vi "AUTON_Index.vi"(0 "Auton Array":dbl[][](array[numeric]), 5 "MeasuredHeading":dbl, 7 "LeftEncoder":dbl, 9 "RightEncoder":dbl) -> ()   [LabVIEW 2012]
uses:
  Robot Global Data.vi
panel:
  out "Right Kicker":dbl
  out "Left Flipper":dbl
  out "Right Flipper":dbl
  out "Shooter Wheel B":dbl
  out "Shooter Wheel F":dbl
  out "Shooter Elevation":dbl
  out "Left Kicker":dbl
  out "Right Drive":dbl
  out "Left Drive":dbl
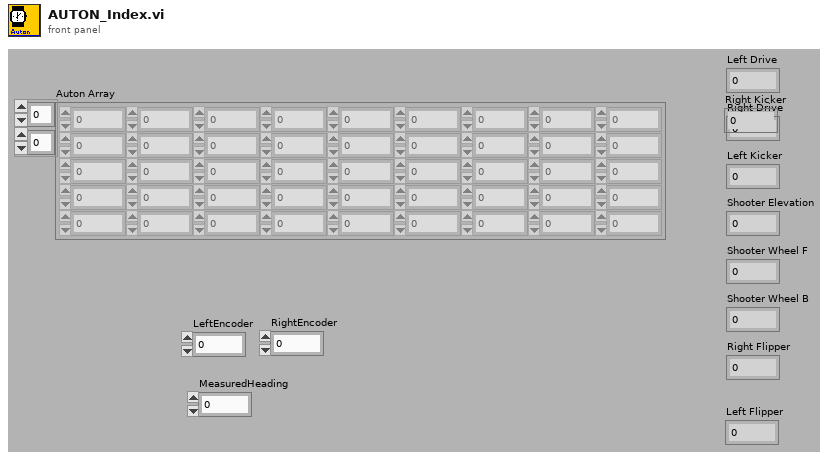
[diagram p1: front panel]
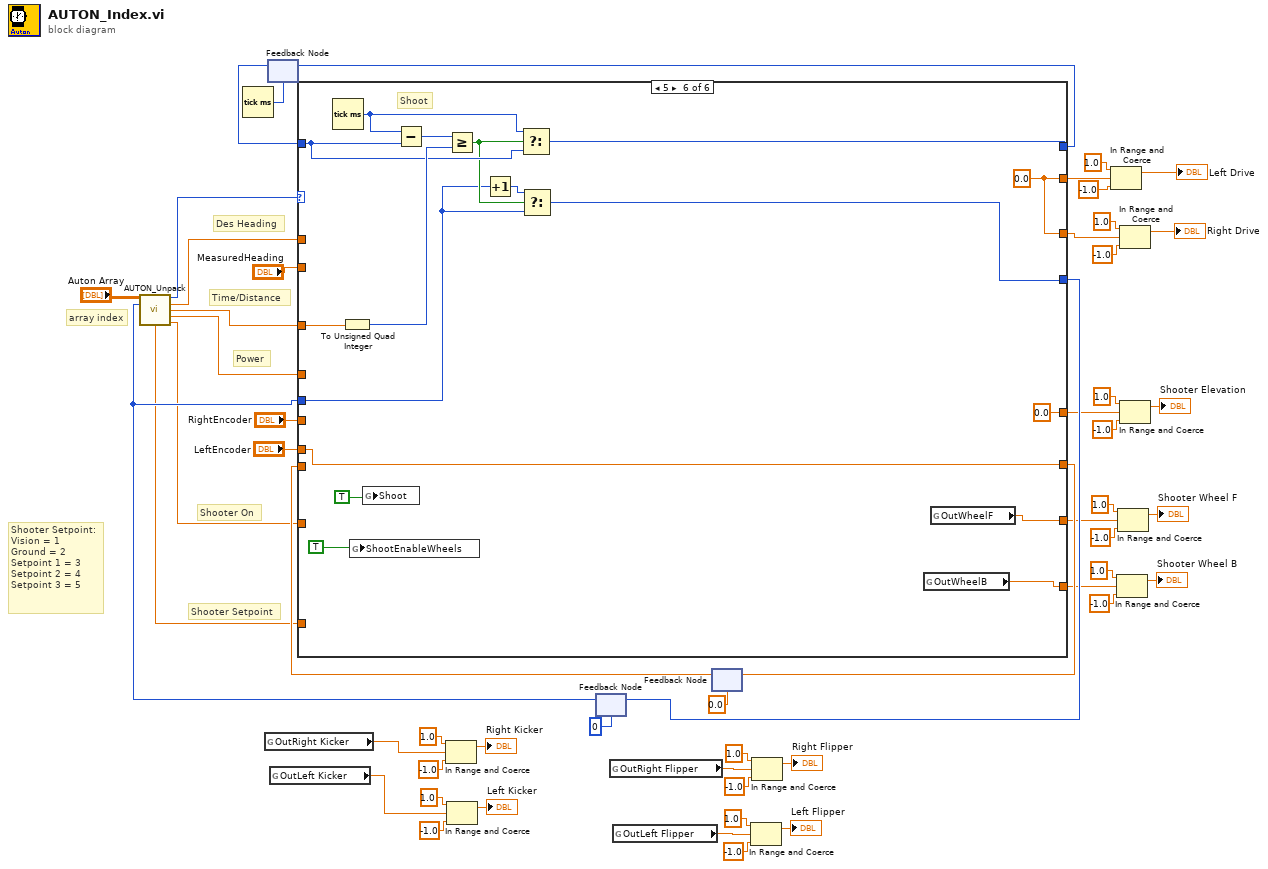
[diagram p0: block diagram]
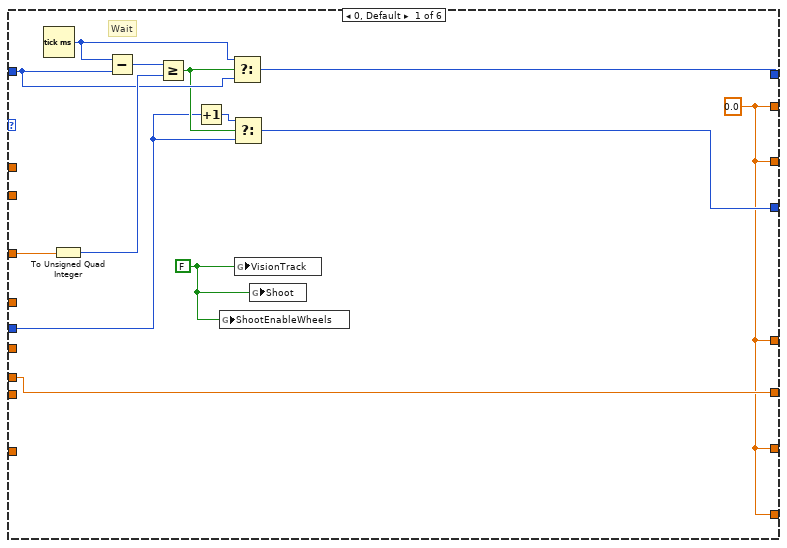
[diagram p2: hidden frame]
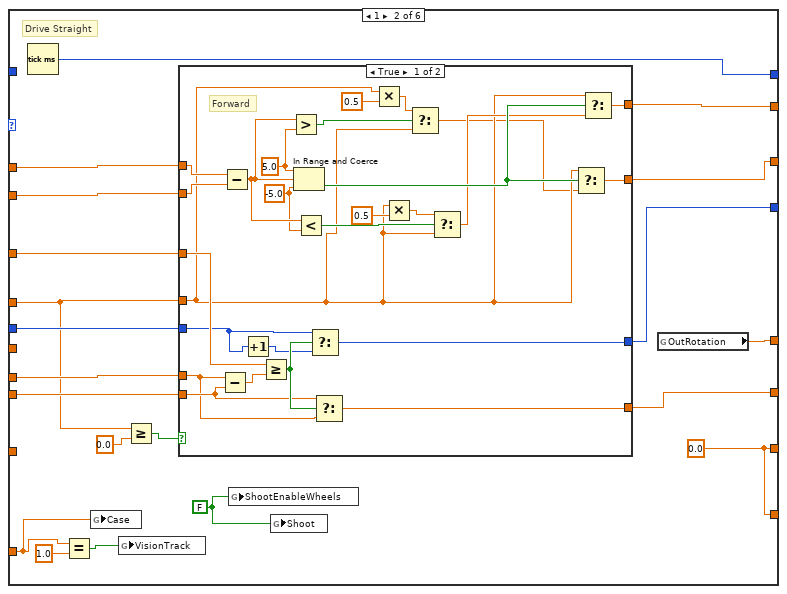
[diagram p3: hidden frame]
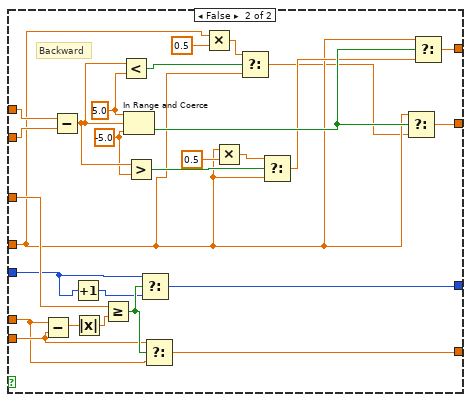
[diagram p4: hidden frame]
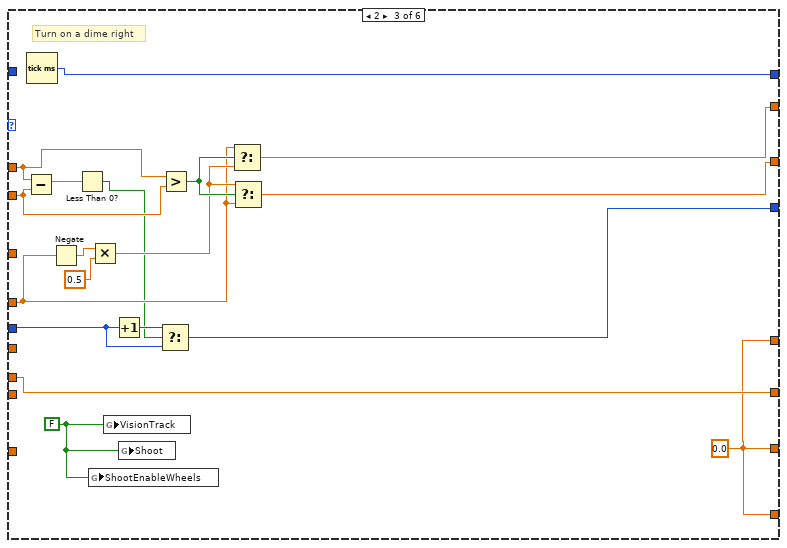
[diagram p5: hidden frame]
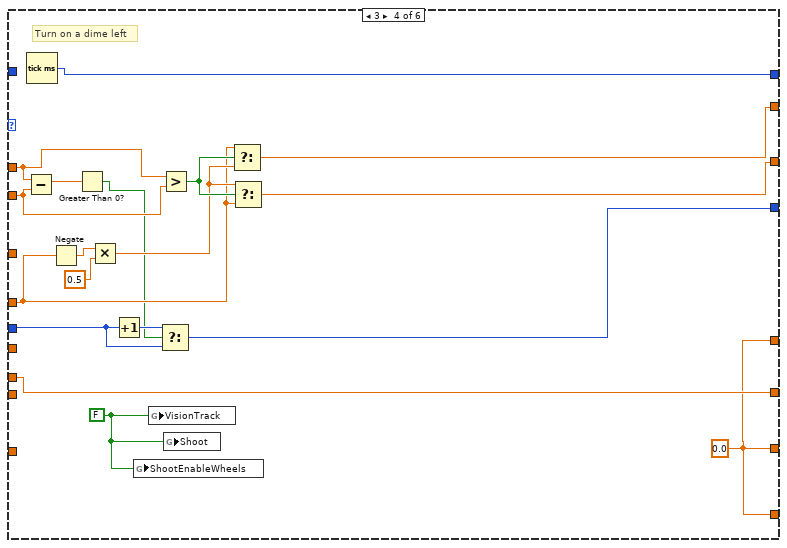
[diagram p6: hidden frame]
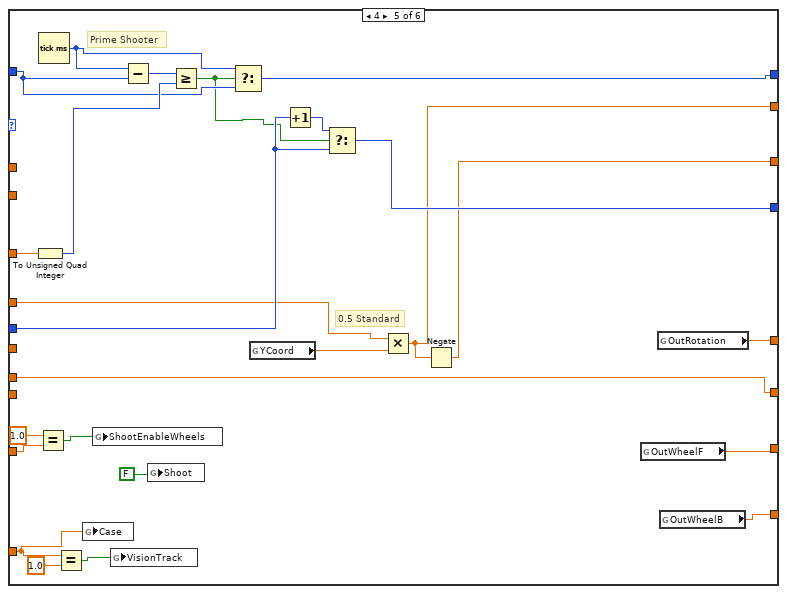
[diagram p7: hidden frame]
diagram:
  # "Shooter Setpoint:\nVision = 1\nGround = 2\nSetpoint 1 = 3\nSetpoint 2 = 4\nSetpoint 3 = 5"
  # "Shooter On"
  # "Shooter Setpoint"
  # "Des Heading"
  # "Time/Distance"
  # "Power"
  # "array index"
  n1 = Tick Count (ms)() -> (millisecond timer value=w52:u32)
  n2 = global read "Robot Global Data.vi" "OutRight Kicker"() -> (w1:dbl)
  n3 = feedback #1(w52) -> (w54:u32)
  n4 = global read "Robot Global Data.vi" "OutLeft Kicker"() -> (w2:dbl)
  n5 = In Range and Coerce(upper limit=1.0, x=w1, lower limit=-1.0) -> (coerced(x)=→"Right Kicker":dbl)  [unwired: 1 out]
  n6 = In Range and Coerce(upper limit=1.0, x=w2, lower limit=-1.0) -> (coerced(x)=→"Left Kicker":dbl)  [unwired: 1 out]
  n7 = feedback #2(0) -> (w31:i32)
  n8 = call "AUTON_Unpack.vi"("all rows"="Auton Array", "Index"=w31) -> ("Primitive ID"=w35:i16, "Desired Heading"=w33:dbl, "Time/Distance"=w32:dbl, "Power"=w34:dbl, "Shooter Setpoint"=w29:dbl, "Shooter Speed"=w30:dbl)  [unwired: 6 in, 2 out]
  n9 = global read "Robot Global Data.vi" "OutRight Flipper"() -> (w10:dbl)
  n10 = global read "Robot Global Data.vi" "OutLeft Flipper"() -> (w9:dbl)
  n11 = feedback #3(0.0) -> (w37:dbl)
  n12 = case shown="5" w35 {
    tunnel: [w60 w86 w154 w172 w201 w211] -> w40
    tunnel: w31 -> [w61 w81 w157 w175 w192 w212]
    tunnel: [w68 w78 w159 w177 w190 w219] -> w42
    tunnel: w54 -> [w65 _ _ _ w191 w216]
    tunnel: w32 -> [w59 w87 _ _ w193 w210]
    tunnel: w33 -> [_ w85 w152 w170 _ _]
    tunnel: [w56 w83 w155 w173 w186 w209] -> w50
    tunnel: [w56 w82 w156 w174 w185 w209] -> w43
    tunnel: w34 -> [_ w77 w146 w164 w187 _]
    tunnel: "LeftEncoder" -> [w57 w79 w153 w171 w202 w207]
    tunnel: "MeasuredHeading" -> [_ w84 w151 w169 _ _]
    tunnel: "RightEncoder" -> [_ _ _ _ _ _]
    tunnel: w37 -> [_ w80 _ _ _ _]
    tunnel: [w57 w88 w153 w171 w202 w207] -> w36
    tunnel: w30 -> [_ _ _ _ w182 _]
    tunnel: w29 -> [_ w71 _ _ w197 _]
    tunnel: [w56 w69 w143 w160 w178 w203] -> w13
    tunnel: [w56 w69 w143 w160 w179 w204] -> w12
    tunnel: [w56 w70 w143 w160 w189 0.0 ("ShootOutElev")] -> w11
    frame 0, Default {
      w58 = FALSE ("ShootTrackEnable")
      w56 = 0.0 ("Numeric")
      # "Wait"
      n13 = Tick Count (ms)() -> (millisecond timer value=w64:u32)
      n14 = To Unsigned Quad Integer(1:w59) -> (0:w66:u64)
      n15 = Subtract(x=w64, y=w65) -> (x-y=w67:u32)
      n16 = Greater Or Equal?(x=w67, y=w66) -> (x >= y?=w63:bool)
      n17 = Increment(x=w61) -> (x+1=w62:i32)
      n18 = global write "Robot Global Data.vi" "ShootEnableWheels"(w58) -> ()
      n19 = Select(t=w64, s=w63, f=w65) -> (s? t:f=w68:u32)
      n20 = Select(t=w62, s=w63, f=w61) -> (s? t:f=w60:i32)
      n21 = global write "Robot Global Data.vi" "VisionTrack"(w58) -> ()
      n22 = global write "Robot Global Data.vi" "Shoot"(w58) -> ()
    }
    frame 1 {
      w74 = FALSE ("ShootTrackEnable")
      w69 = 0.0 ("Numeric")
      # "Drive Straight"
      n23 = Tick Count (ms)() -> (millisecond timer value=w78:u32)
      n24 = Equal?(x=w71, y=1.0) -> (x = y?=w72:bool)
      n25 = global write "Robot Global Data.vi" "Case"(w71) -> ()
      n26 = global write "Robot Global Data.vi" "VisionTrack"(w72) -> ()
      n27 = Greater Or Equal?(x=w77, y=0.0) -> (x >= y?=w75:bool)
      n28 = case shown="True" w75 {
        tunnel: [w114 w141] -> w88
        tunnel: w87 -> [w112 w140]
        tunnel: [w110 w138] -> w86
        tunnel: w85 -> [w109 w137]
        tunnel: w84 -> [w108 w136]
        tunnel: [w106 w134] -> w83
        tunnel: [w105 w133] -> w82
        tunnel: w77 -> [w94 w122]
        tunnel: w81 -> [w91 w119]
        tunnel: w80 -> [w90 w118]
        tunnel: w79 -> [w89 w117]
        frame True {
          w102 = -5.0 ("lower limit")
          w104 = 5.0 ("upper limit")
          # "Forward"
          n29 = Subtract(x=w89, y=w90) -> (x-y=w113:dbl)
          n30 = Subtract(x=w109, y=w108) -> (x-y=w103:dbl)
          n31 = Increment(x=w91) -> (x+1=w92:i32)
          n32 = Greater Or Equal?(x=w112, y=w113) -> (x >= y?=w111:bool)
          n33 = Greater?(x=w103, y=w104) -> (0:w97:bool)
          n34 = In Range and Coerce(upper limit=w104, x=w103, lower limit=w102) -> (In Range?=w107:bool)  [unwired: 1 out]
          n35 = Less?(x=w103, y=w102) -> (x < y?=w101:bool)
          n36 = Select(t=w91, s=w111, f=w92) -> (s? t:f=w110:i32)
          n37 = Select(t=w90, s=w111, f=w89) -> (s? t:f=w114:dbl)
          n38 = Multiply(x=w94, y=0.5) -> (x*y=w96:dbl)
          n39 = Multiply(x=w94, y=0.5) -> (x*y=w99:dbl)
          n40 = Select(t=w96, s=w97, f=w94) -> (s? t:f=w93:dbl)
          n41 = Select(t=w99, s=w101, f=w94) -> (s? t:f=w98:dbl)
          n42 = Select(t=w94, s=w107, f=w93) -> (s? t:f=w105:dbl)
          n43 = Select(t=w94, s=w107, f=w98) -> (s? t:f=w106:dbl)
        }
        frame False {
          w130 = -5.0 ("lower limit")
          w132 = 5.0 ("upper limit")
          # "Backward"
          n44 = Subtract(x=w117, y=w118) -> (x-y=w115:dbl)
          n45 = Subtract(x=w137, y=w136) -> (x-y=w131:dbl)
          n46 = Increment(x=w119) -> (x+1=w120:i32)
          n47 = Absolute Value(x=w115) -> (abs(x)=w116:dbl)
          n48 = Greater Or Equal?(x=w140, y=w116) -> (x >= y?=w139:bool)
          n49 = Less?(x=w131, y=w132) -> (x < y?=w125:bool)
          n50 = In Range and Coerce(upper limit=w132, x=w131, lower limit=w130) -> (In Range?=w135:bool)  [unwired: 1 out]
          n51 = Greater?(x=w131, y=w130) -> (0:w129:bool)
          n52 = Select(t=w119, s=w139, f=w120) -> (s? t:f=w138:i32)
          n53 = Select(t=w118, s=w139, f=w117) -> (s? t:f=w141:dbl)
          n54 = Multiply(x=w122, y=0.5) -> (x*y=w124:dbl)
          n55 = Multiply(x=w122, y=0.5) -> (x*y=w127:dbl)
          n56 = Select(t=w124, s=w125, f=w122) -> (s? t:f=w121:dbl)
          n57 = Select(t=w127, s=w129, f=w122) -> (s? t:f=w126:dbl)
          n58 = Select(t=w122, s=w135, f=w121) -> (s? t:f=w133:dbl)
          n59 = Select(t=w122, s=w135, f=w126) -> (s? t:f=w134:dbl)
        }
      }
      n60 = global write "Robot Global Data.vi" "ShootEnableWheels"(w74) -> ()
      n61 = global write "Robot Global Data.vi" "Shoot"(w74) -> ()
      n62 = global read "Robot Global Data.vi" "OutRotation"() -> (w70:dbl)
    }
    frame 2 {
      w142 = FALSE ("ShootTrackEnable")
      w143 = 0.0 ("Numeric")
      # "Turn on a dime right"
      n63 = Subtract(x=w152, y=w151) -> (x-y=w145:dbl)
      n64 = Tick Count (ms)() -> (millisecond timer value=w159:u32)
      n65 = Negate(x=w146) -> (-x=w149:dbl)
      n66 = Less Than 0?(x=w145) -> (x < 0?=w144:bool)
      n67 = global write "Robot Global Data.vi" "ShootEnableWheels"(w142) -> ()
      n68 = Multiply(x=w149, y=0.5) -> (x*y=w147:dbl)
      n69 = global write "Robot Global Data.vi" "VisionTrack"(w142) -> ()
      n70 = Increment(x=w157) -> (x+1=w158:i32)
      n71 = global write "Robot Global Data.vi" "Shoot"(w142) -> ()
      n72 = Select(t=w158, s=w144, f=w157) -> (s? t:f=w154:i32)
      n73 = Greater?(x=w152, y=w151) -> (0:w150:bool)
      n74 = Select(t=w146, s=w150, f=w147) -> (s? t:f=w155:dbl)
      n75 = Select(t=w147, s=w150, f=w146) -> (s? t:f=w156:dbl)
    }
    frame 3 {
      w161 = FALSE ("ShootTrackEnable")
      w160 = 0.0 ("Numeric")
      # "Turn on a dime left"
      n76 = Subtract(x=w170, y=w169) -> (x-y=w163:dbl)
      n77 = Tick Count (ms)() -> (millisecond timer value=w177:u32)
      n78 = Negate(x=w164) -> (-x=w167:dbl)
      n79 = Greater Than 0?(x=w163) -> (x > 0?=w162:bool)
      n80 = Multiply(x=w167, y=0.5) -> (x*y=w165:dbl)
      n81 = Increment(x=w175) -> (x+1=w176:i32)
      n82 = global write "Robot Global Data.vi" "ShootEnableWheels"(w161) -> ()
      n83 = global write "Robot Global Data.vi" "VisionTrack"(w161) -> ()
      n84 = Select(t=w176, s=w162, f=w175) -> (s? t:f=w172:i32)
      n85 = Greater?(x=w170, y=w169) -> (0:w168:bool)
      n86 = global write "Robot Global Data.vi" "Shoot"(w161) -> ()
      n87 = Select(t=w164, s=w168, f=w165) -> (s? t:f=w173:dbl)
      n88 = Select(t=w165, s=w168, f=w164) -> (s? t:f=w174:dbl)
    }
    frame 4 {
      # "0.5 Standard"
      # "Prime Shooter"
      n89 = To Unsigned Quad Integer(1:w193) -> (0:w195:u64)
      n90 = Equal?(x=1.0, y=w182) -> (x = y?=w180:bool)
      n91 = Tick Count (ms)() -> (millisecond timer value=w194:u32)
      n92 = Equal?(x=w197, y=1.0) -> (x = y?=w198:bool)
      n93 = global write "Robot Global Data.vi" "Case"(w197) -> ()
      n94 = global write "Robot Global Data.vi" "ShootEnableWheels"(w180) -> ()
      n95 = global write "Robot Global Data.vi" "VisionTrack"(w198) -> ()
      n96 = Subtract(x=w194, y=w191) -> (x-y=w196:u32)
      n97 = global write "Robot Global Data.vi" "Shoot"(FALSE ("Shoot")) -> ()
      n98 = Greater Or Equal?(x=w196, y=w195) -> (x >= y?=w188:bool)
      n99 = Select(t=w194, s=w188, f=w191) -> (s? t:f=w190:u32)
      n100 = global read "Robot Global Data.vi" "YCoord"() -> (w184:dbl)
      n101 = Increment(x=w192) -> (x+1=w200:i32)
      n102 = Select(t=w200, s=w188, f=w192) -> (s? t:f=w201:i32)
      n103 = Multiply(x=w187, y=w184) -> (x*y=w186:dbl)
      n104 = Negate(x=w186) -> (-x=w185:dbl)
      n105 = global read "Robot Global Data.vi" "OutWheelF"() -> (w179:dbl)
      n106 = global read "Robot Global Data.vi" "OutRotation"() -> (w189:dbl)
      n107 = global read "Robot Global Data.vi" "OutWheelB"() -> (w178:dbl)
    }
    frame 5 {
      w209 = 0.0 ("Numeric")
      # "Shoot"
      n108 = Tick Count (ms)() -> (millisecond timer value=w215:u32)
      n109 = To Unsigned Quad Integer(1:w210) -> (0:w217:u64)
      n110 = global write "Robot Global Data.vi" "ShootEnableWheels"(TRUE ("ShootEnableWheels")) -> ()
      n111 = global write "Robot Global Data.vi" "Shoot"(TRUE ("Shoot")) -> ()
      n112 = Subtract(x=w215, y=w216) -> (x-y=w218:u32)
      n113 = Greater Or Equal?(x=w218, y=w217) -> (x >= y?=w214:bool)
      n114 = Increment(x=w212) -> (x+1=w213:i32)
      n115 = Select(t=w215, s=w214, f=w216) -> (s? t:f=w219:u32)
      n116 = Select(t=w213, s=w214, f=w212) -> (s? t:f=w211:i32)
      n117 = global read "Robot Global Data.vi" "OutWheelB"() -> (w203:dbl)
      n118 = global read "Robot Global Data.vi" "OutWheelF"() -> (w204:dbl)
    }
  }
  n119 = feedback-in #1(w42) -> ()
  n120 = feedback-in #2(w40) -> ()
  n121 = feedback-in #3(w36) -> ()
  n122 = In Range and Coerce(upper limit=1.0, x=w9, lower limit=-1.0) -> (coerced(x)=→"Left Flipper":dbl)  [unwired: 1 out]
  n123 = In Range and Coerce(upper limit=1.0, x=w10, lower limit=-1.0) -> (coerced(x)=→"Right Flipper":dbl)  [unwired: 1 out]
  n124 = In Range and Coerce(upper limit=1.0, x=w50, lower limit=-1.0) -> (coerced(x)=→"Left Drive":dbl)  [unwired: 1 out]
  n125 = In Range and Coerce(upper limit=1.0, x=w13, lower limit=-1.0) -> (coerced(x)=→"Shooter Wheel B":dbl)  [unwired: 1 out]
  n126 = In Range and Coerce(upper limit=1.0, x=w12, lower limit=-1.0) -> (coerced(x)=→"Shooter Wheel F":dbl)  [unwired: 1 out]
  n127 = In Range and Coerce(upper limit=1.0, x=w43, lower limit=-1.0) -> (coerced(x)=→"Right Drive":dbl)  [unwired: 1 out]
  n128 = In Range and Coerce(upper limit=1.0, x=w11, lower limit=-1.0) -> (coerced(x)=→"Shooter Elevation":dbl)  [unwired: 1 out]
